vi "7- Greater than 30 in an array.vi"() -> ()   [LabVIEW 2019]
panel:
  in  "?":bool
  out "?":i32
  out "?":dbl[](array[numeric]) format="%#_3g"
  # "First index in the array of Random number that have a number greater than 30."
  # "** Index 8 depict overflow that means number greater than 30 is not present in array."
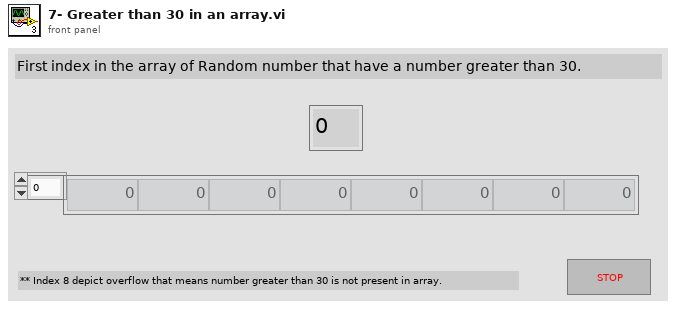
[diagram p1: front panel]
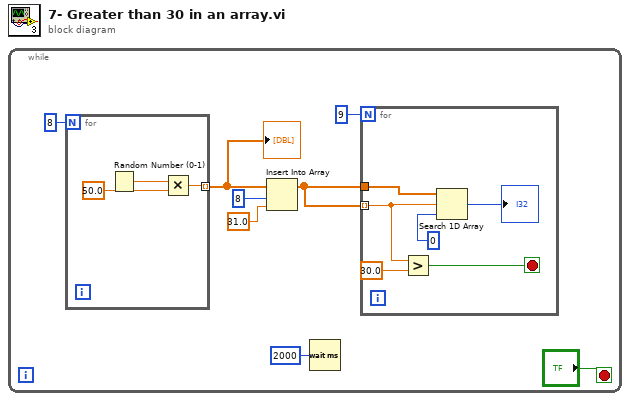
[diagram p0: block diagram]
diagram:
  n1 = while {
    stop <- "?" stop-if-true
    n2 = for {
      N: 8 -> [_]
      tunnel: [w15] -> w1 mode=indexing
      n3 = Random Number (0-1)() -> (number: 0 to 1=w17:dbl)
      n4 = Multiply(x=w17, y=50.0) -> (x*y=w15:dbl)
    }
    "?" <- w1
    n5 = Insert Into Array(array=w1, index=8, new element=31.0 ("new element/subarray")) -> (w4:dbl[])
    n6 = Wait (ms)(milliseconds to wait=u32 2000) -> ()  [unwired: 1 out]
    n7 = for {
      N: 9 -> [_]
      tunnel: w4 -> [w11] mode=indexing
      tunnel: w4 -> [w12]
      stop <- w9 stop-if-true
      n8 = Greater?(x=w11, y=30.0) -> (0:w9:bool)
      n9 = Search 1D Array(1D array=w12, element=w11, start index (0)=0) -> (index of element=→"?":i32)
    }
  }
